vi "calculateJumperRiseAndFallTime-v03.vi"(8 "jumptestMonitor":waveform(dbl)(graph)={"t0"=timestamp(3645557132.4115305 s since 1904-01-01), "dt"=4.999999999999997e-05, "Y"=array[200000 elements], "attributes"=variant("NI_ChannelName"=variant(string "AI-jump"), "NI_UnitDescription"=variant(string "Volts"))}, 11 "output cluster":T1={"daq_ao 2"="Dev1/ao1", "Duration (s)"=10.0, "Sample Freq (Hz)"=20000.0, "Phase"=-36.0, "duty cycle"=10.0, "Jump Filter Freq (Hz)"=30.0, "Number of Replicates"=1} {"Number of Replicates" min=1 max=10}) -> (1 "fall time (ms)":dbl, 2 "rise time (ms)":dbl)   [LabVIEW 2015]
uses:
  <vilib>/Analysis/NI_AALBase.lvlib
  <vilib>/Analysis/baseanly.llb/Mean (DBL).vi
panel:
  out "fall clip":waveform(dbl)(graph)={"t0"=timestamp(3645557132.4115305 s since 1904-01-01), "dt"=4.999999999999997e-05, "Y"=array[6001 elements], "attributes"=variant("NI_ChannelName"=variant(string "AI-jump"), "NI_UnitDescription"=variant(string "Volts"))} caption="jumptestMonitor"
  out "rise clip":waveform(dbl)(graph)={"t0"=timestamp(3645557132.4115305 s since 1904-01-01), "dt"=4.999999999999997e-05, "Y"=array[6001 elements], "attributes"=variant("NI_ChannelName"=variant(string "AI-jump"), "NI_UnitDescription"=variant(string "Volts"))} caption="jumptestMonitor"
  out "full wave":waveform(dbl)(graph)={"t0"=timestamp(3645557132.4115305 s since 1904-01-01), "dt"=4.999999999999997e-05, "Y"=array[200000 elements], "attributes"=variant("NI_ChannelName"=variant(string "AI-jump"), "NI_UnitDescription"=variant(string "Volts"))} caption="jumptestMonitor"
  out "full rise calc":dbl
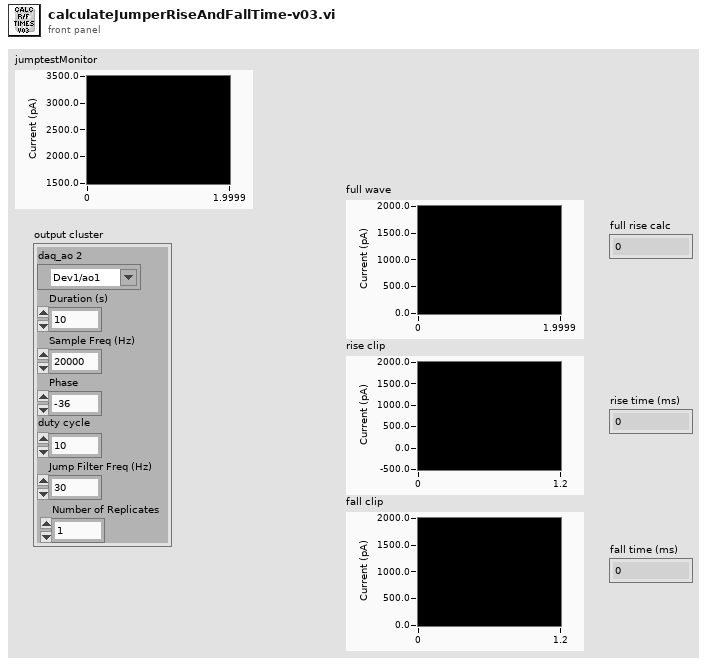
[diagram p1: front panel]
types:
  T1 = cluster{"daq_ao 2":tag, "Duration (s)":dbl, "Sample Freq (Hz)":dbl, "Phase":dbl, "duty cycle":dbl, "Jump Filter Freq (Hz)":dbl, "Number of Replicates":i16}
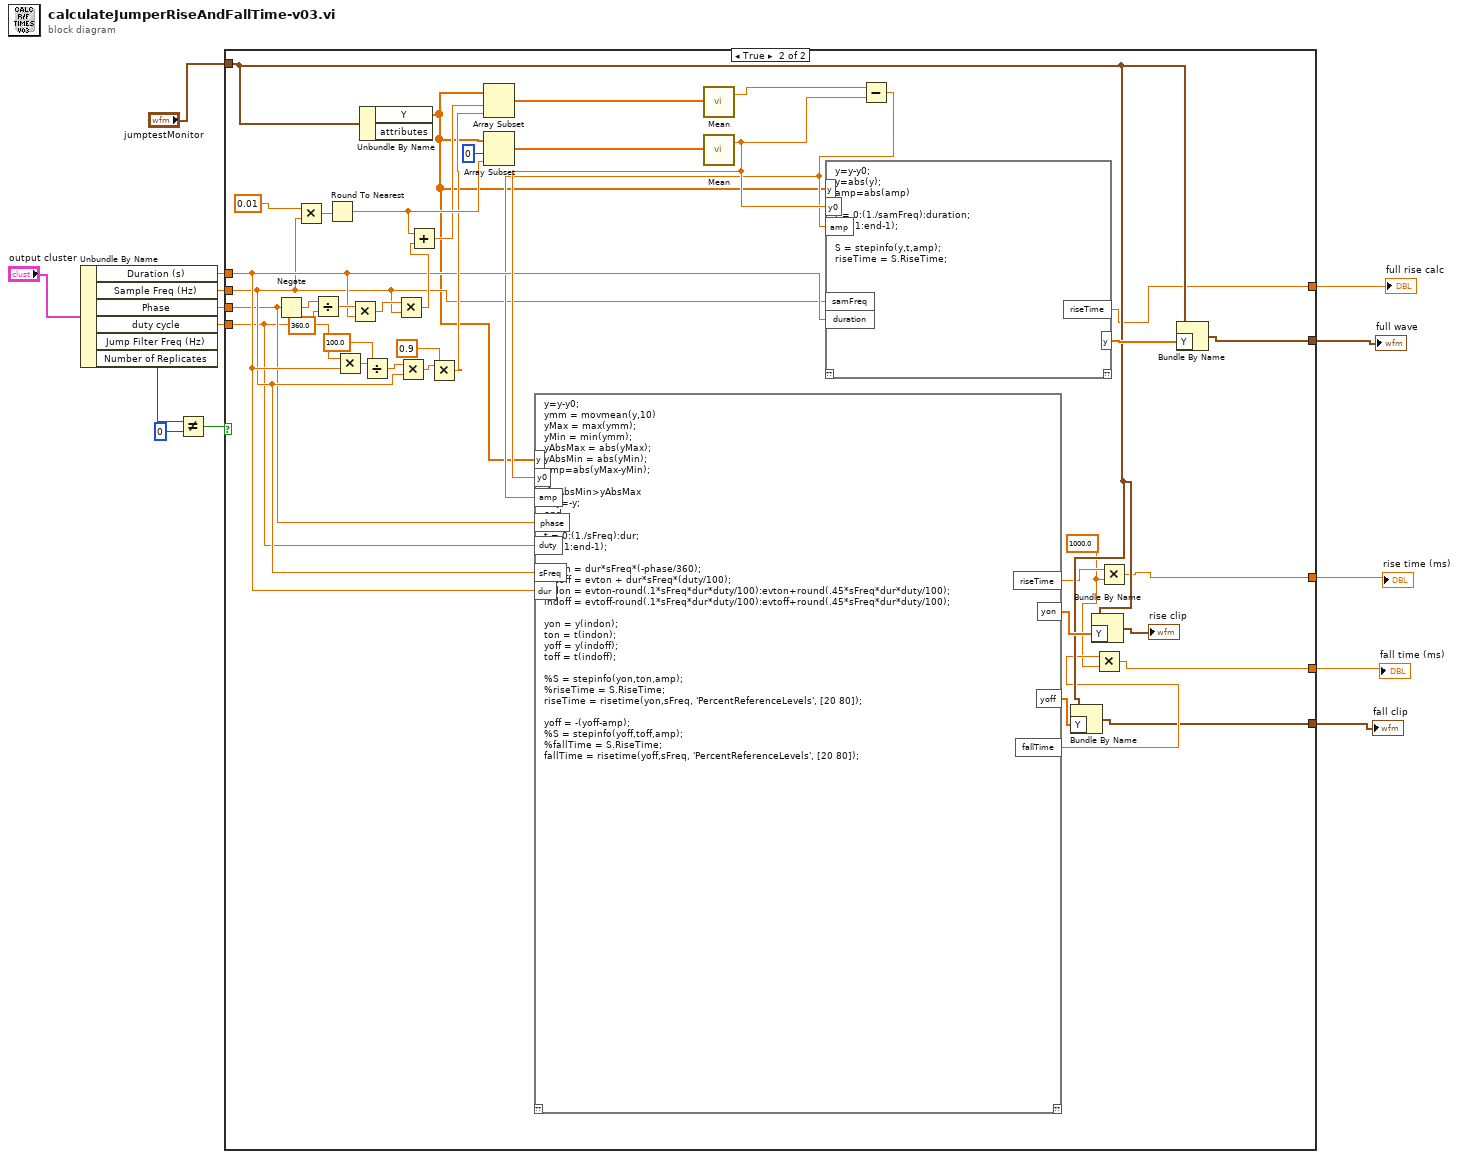
[diagram p0: block diagram]
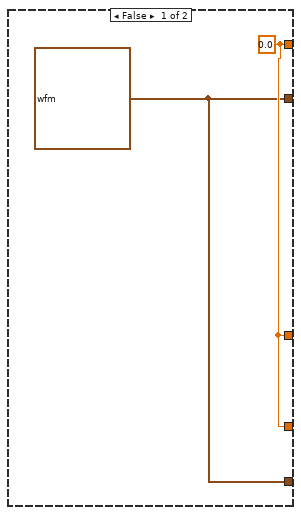
[diagram p2: hidden frame]
diagram:
  n1 = Unbundle By Name("output cluster") -> ("Duration (s)"=w13:dbl, "Sample Freq (Hz)"=w11:dbl, "Phase"=w10:dbl, "duty cycle"=w9:dbl, "Number of Replicates"=w7:i16)  [unwired: 1 out]
  n2 = Not Equal?(x=w7, y=i16 0) -> (x != y?=w8:bool)
  n3 = case shown="True" w8 {
    tunnel: w13 -> [_ w34]
    tunnel: "jumptestMonitor" -> [_ w31]
    tunnel: w11 -> [_ w29]
    tunnel: w10 -> [_ w27]
    tunnel: w9 -> [_ w26]
    tunnel: [w16 w21] -> w5
    tunnel: [w16 w20] -> w4
    tunnel: [w15 w19] -> w3
    tunnel: [w16 w18] -> w2
    tunnel: [w15 w17] -> w1
    frame False {
      w15 = waveform(dbl) {"t0"=timestamp(0 s since 1904-01-01), "dt"=1.0, "Y"=[]} ("jumptestMonitor")
      w16 = 0.0
    }
    frame True {
      w22 = 1000.0 ("y")
      n4 = Negate(x=w27) -> (-x=w49:dbl)
      n5 = Multiply(x=0.01, y=w29) -> (x*y=w53:dbl)
      n6 = Divide(x=w49, y=360.0) -> (x/y=w47:dbl)
      n7 = Round To Nearest(number=w53) -> (nearest integer value=w40:dbl)
      n8 = Multiply(x=w26, y=w34) -> (x*y=w45:dbl)
      n9 = Multiply(x=w47, y=w34) -> (x*y=w46:dbl)
      n10 = Unbundle By Name(w31) -> ("Y"=w28:dbl[])  [unwired: 1 out]
      n11 = Divide(x=w45, y=100.0) -> (x/y=w43:dbl)
      n12 = Multiply(x=w46, y=w29) -> (x*y=w41:dbl)
      n13 = Multiply(x=w43, y=w29) -> (x*y=w37:dbl)
      n14 = Add(x=w40, y=w41) -> (x+y=w39:dbl)
      n15 = Multiply(x=w37, y=0.9) -> (x*y=w38:dbl)
      n16 = Array Subset(array=w28, index=w39, length=w38) -> (w51:dbl[])
      n17 = Array Subset(array=w28, index=0, length=w40) -> (w52:dbl[])
      n18 = call-poly <vilib>:"Mean.vi"("X"=w51) -> ("mean"=w50:dbl)  [unwired: 1 out]
      n19 = call-poly <vilib>:"Mean.vi"("X"=w52) -> ("mean"=w35:dbl)  [unwired: 1 out]
      n20 = Subtract(x=w50, y=w35) -> (x-y=w30:dbl)
      n21 = script code="y=y-y0;\nymm = movmean(y,10)\nyMax = max(ymm);\nyMin = min(ymm);\nyAbsMax = abs(yMax);\nyAbsMin = abs(yMin);\namp=abs(yMax-yMin);\n\nif yAbsMin>yAbsMax\n    y=-y;\nend\n\nt = 0:(1./sFreq):dur;\nt=t(1:end-1);\n\nevton = dur*sFreq*(-phase/360);\nevtoff = evton + dur*sFreq*(duty/100);\nindon = evton-round(.1*sFreq*dur*duty/100):evton+round(.45*sFreq*dur*duty/100);\nindoff = evtoff-round(.1*sFreq*dur*duty/100):evtoff+round(.45*sFreq*dur*duty/100);\n\nyon = y(indon);\nton = t(indon);\nyoff = y(indoff);\ntoff = t(indoff);\n\n%S = stepinfo(yon,ton,amp);\n%riseTime = S.RiseTime;\nriseTime = risetime(yon,sFreq, 'PercentReferenceLevels', [20 80]);\n\nyoff = -(yoff-amp);\n%S = stepinfo(yoff,toff,amp);\n%fallTime = S.RiseTime;\nfallTime = risetime(yoff,sFreq, 'PercentReferenceLevels', [20 80]);"("y"=w28, "sFreq"=w29, "dur"=w34, "y0"=w35, "amp"=w30, "phase"=w27, "duty"=w26) -> ("riseTime"=w24:dbl, "yon"=w32:dbl[], "yoff"=w25:dbl[], "fallTime"=w23:dbl)  [unwired: 1 in, 1 out]
      n22 = script code="y=y-y0;\ny=abs(y);\namp=abs(amp)\n\nt = 0:(1./samFreq):duration;\nt=t(1:end-1);\n\nS = stepinfo(y,t,amp);\nriseTime = S.RiseTime;"("y"=w28, "samFreq"=w29, "duration"=w34, "y0"=w35, "amp"=w30) -> ("riseTime"=w18:dbl, "y"=w42:dbl[])  [unwired: 1 in, 1 out]
      n23 = Bundle By Name(cluster=w31, "Y"=w25) -> (w17:waveform(dbl))
      n24 = Bundle By Name(cluster=w31, "Y"=w32) -> (→"rise clip":waveform(dbl))
      n25 = Multiply(x=w23, y=w22) -> (x*y=w21:dbl)
      n26 = Multiply(x=w24, y=w22) -> (x*y=w20:dbl)
      n27 = Bundle By Name(cluster=w31, "Y"=w42) -> (w19:waveform(dbl))
    }
  }
  "fall time (ms)" <- w5
  "rise time (ms)" <- w4
  "full wave" <- w3
  "full rise calc" <- w2
  "fall clip" <- w1
